vi "Firmware.vi"() -> ()   [LabVIEW 2017]
uses:
  <vilib>/Platform/TimedLoop/XDataNode/timing_clust.ctl
  <vilib>/Platform/TimedLoop/XDataNode/nitl_modes.ctl
  <vilib>/Platform/TimedLoop/XDataNode/wakeup.ctl
  <instrlib>/_niInstr/Instruction Framework/v1/FPGA/Helper Classes/Single Address Space Collection/Single Address Space Collection.lvclass
  C:/Program Files (x86)/National Instruments/LabVIEW 2017/instr.lib/_niInstr/Instruction Framework/v1/FPGA/Interfaces/Address Space Collection/Address Space Collection.lvclass
  <instrlib>/_niInstr/FIFO Register Bus/v1/FPGA/niInstr FIFO Register Bus v1 FPGA.lvclass
  C:/Program Files (x86)/National Instruments/LabVIEW 2017/instr.lib/_niInstr/Instruction Framework/v1/FPGA/Interfaces/Instruction Producer/Instruction Producer.lvclass
  <vilib>/rvi/Emulation/niFpgaGetClockAttributes.vi
  <vilib>/rvi/Emulation/niFpgaSctlEmulationGetInTimedLoop.vi
  <vilib>/rvi/Emulation/niFpgaEmulationReportErrorSimple.vi
  <vilib>/rvi/Emulation/niFpgaProcessEmulError.vi
  <vilib>/rvi/Emulation/niFpgaCriticalErrorInLSC.vi
  <vilib>/rvi/eio/common/nirviEmuTemplateMethod_errors.vi
  <vilib>/eio/EIONode/EIONode.xnode
  <vilib>/Platform/TimedLoop/XDataNode/XDataNode.xnode
  <instrlib>/_niInstr/Instruction Framework/v1/FPGA/Top Level Bus/Register Configuration/Register Configuration.lvclass
  <vilib>/Platform/TimedLoop/XDataNode/XDNodeRunTimeDep.lvlib
  <vilib>/NI/PowerElectronicsControl/ScaleAndLimit/Core/ScaleAndLimit.lvlib
  <vilib>/NI/PowerElectronicsControl/ScaleAndLimit/Core/AddressSpace.lvclass
  <vilib>/NI/PowerElectronicsControl/WaveformAcq/FPGA/WaveformAddressSpace.lvclass
panel:
  out "FaultBuffer":u64 format="%.0x"
  out "LimitsFlag":bool
  out "Sourcing_P1_DI":u16
  out "Sourcing_P0_DI":u16
  out "Sinking_DO":u32 format="%.0x"
  out "Scanned_AI":sgl[](array[numeric])
  out "AO":i16[](array[numeric])
  out "RelayControl_DO":u8 format="%.0x"
  out "LVTTL_DIO":u32 format="%.0x"
  out "HalfBridge":u16 format="%.0x"
  out "TriggerTimestamp":i32
  out "relativeTimestamp":i32
  in  "ManualTrigger":bool
  in  "fifo reg bus ctrl 0":u32
  out "fifo reg bus status 0":u32
  out "fifo reg bus data 0":u64
  out "SimultaneousAILoopRate":u32
  out "Simultaneous_AI":sgl[](array[numeric])
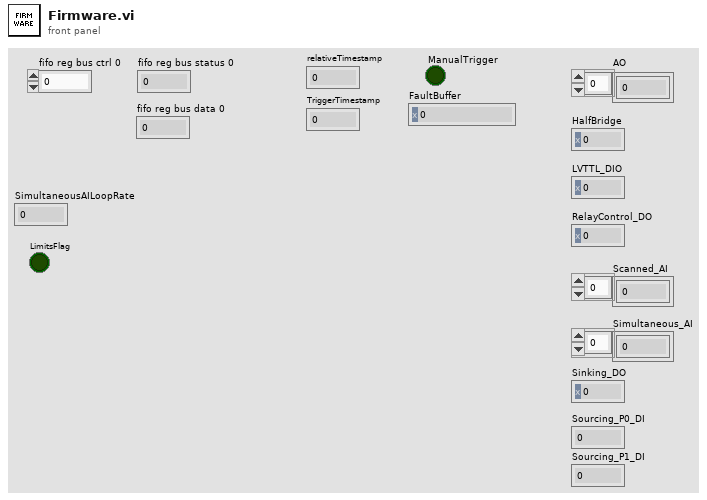
[diagram p1: front panel]
types:
  T1 = typedef "XDNodeRunTimeDep.lvlib/timing_clust.ctl" = cluster{"Expected End [f-1]":u64, "Actual End [f-1]":u64, "Finished Late? [f-1]":bool, "Expected End [i-1]":u64, "Actual End [i-1]":u64, "Finished Late? [i-1]":bool, "Expected Start [i]":u64, "Actual Start [i]":u64, "Expected Start [f]":u64, "Actual Start [f]":u64, "Source Name":string, "Structure Name":string, "Period":i64, "Deadline":i64, "Offset":i64, "Start":i64, "Priority":i32, "Timeout":i32, "Mode":T2, "Wakeup Reason":T3, "Error":errorcluster, "Source Type":string, "Secondary Source Type":string, "Global End Time":u64, "Global Start Time":u64, "Frame Duration":u64, "Iteration Duration":u64, "Assigned CPU":i32, "I/O Scan Engine Mode":u32}
  T2 = typedef "XDNodeRunTimeDep.lvlib/nitl_modes.ctl" = enum32{"No Change", "Process missed periods, maintain original phase", "Discard missed periods, maintain original phase", "Process missed periods, ignore original phase", "Discard missed periods, ignore original phase"}
  T3 = typedef "XDNodeRunTimeDep.lvlib/wakeup.ctl" = enum32{"Normal", "Aborted", "Asynchronous wakeup", "Timing source error", "Timed loop error", "Timeout"}
  T4 = typedef "ScaleAndLimit.lvlib/LimitsRegisters.ctl" = cluster{"HighLimits":refnum<k21>, "LowLimits":refnum<k21>, "ClearLimits":refnum<k21>, "LimitsFlag":refnum<k21>}
  T5 = typedef "ScaleAndLimit.lvlib/ConfigRegisters.ctl" = cluster{"LimitsEnabled":refnum<k21>, "UnscaledHighLimit":refnum<k21>, "UnscaledLowLimit":refnum<k21>, "B":refnum<k21>, "M":refnum<k21>}
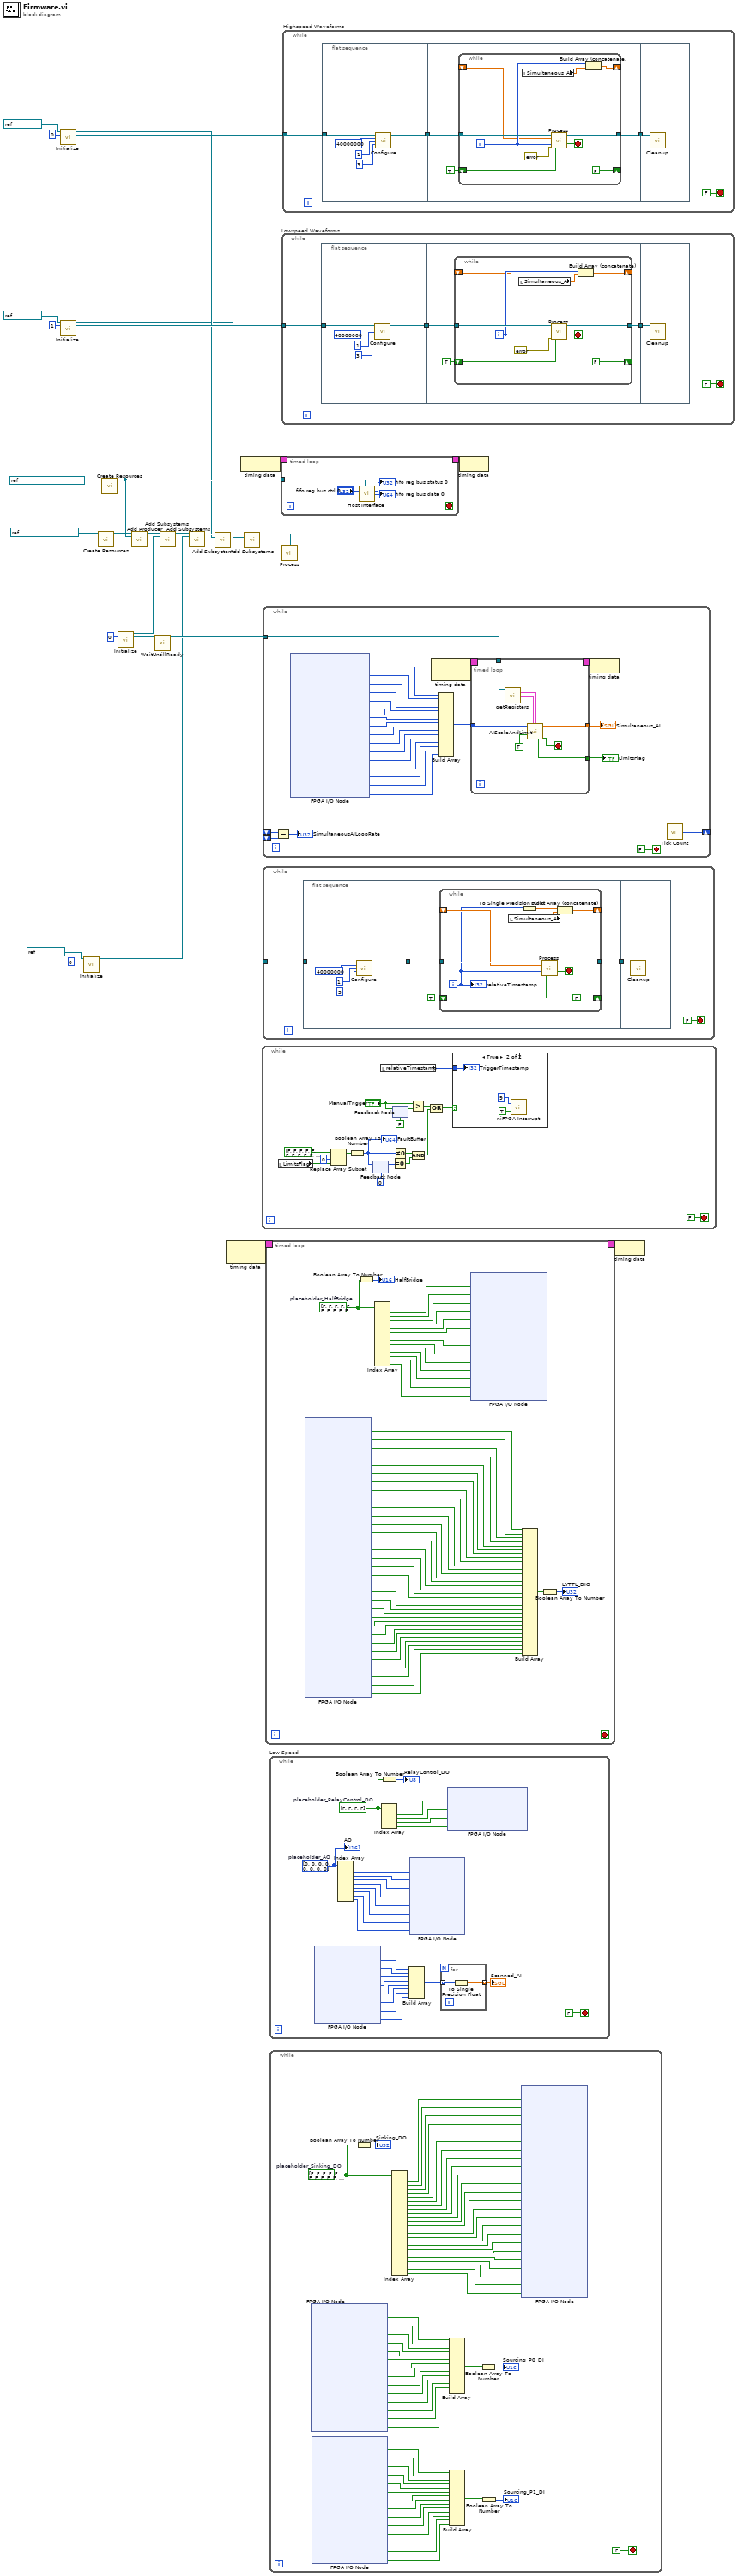
[diagram p0: block diagram]
diagram:
  n1 = call <vilib>:"Initialize.vi"("DMA FIFO"=refnum<k21> "DataSGL0" ("FIFO Out"), "instance"=u8 0) -> ("subsystem"=w3:refnum<class "Single Address Space Collection.lvclass">, "AddressSpace"=w9:refnum<class "WaveformAddressSpace.lvclass">)  [unwired: 12 in]
  n2 = call <vilib>:"Initialize.vi"("DMA FIFO"=refnum<k21> "DataSGL1" ("FIFO Out"), "instance"=u8 1) -> ("subsystem"=w2:refnum<class "Single Address Space Collection.lvclass">, "AddressSpace"=w8:refnum<class "WaveformAddressSpace.lvclass">)  [unwired: 12 in]
  n3 = call <vilib>:"Initialize.vi"("DMA FIFO"=refnum<k21> "DataSGL0" ("FIFO Out"), "instance"=u8 0) -> ("subsystem"=w14:refnum<class "Single Address Space Collection.lvclass">, "AddressSpace"=w16:refnum<class "WaveformAddressSpace.lvclass">)  [unwired: 12 in]
  n4 = call <instrlib>:"Create Resources.vi"("register clock"=refnum<k21> "40 MHz Onboard Clock") -> ("register configuration"=w27:refnum<class "Register Configuration.lvclass">)  [unwired: 14 in]
  n5 = call <instrlib>:"Create Resources.vi"("instruction fifo"=refnum<k21> "reg.host instruction fifo 0") -> ("fifo register bus"=w19:refnum<class "niInstr FIFO Register Bus v1 FPGA.lvclass">)  [unwired: 14 in]
  n6 = call <vilib>:"Initialize.vi"("instance"=u8 0) -> ("subsystem"=w24:refnum<class "Single Address Space Collection.lvclass">, "AddressSpace"=w22:refnum<class "AddressSpace.lvclass">)  [unwired: 13 in]
  n7 = call <instrlib>:"Add Producer.vi"("register configuration in"=w27, "instruction producer"=w19) -> ("register configuration out"=w25:refnum<class "Register Configuration.lvclass">)  [unwired: 13 in]
  n8 = call <vilib>:"WaitUntillReady.vi"("AddressSpace in"=w22) -> ("AddressSpace out"=w21:refnum<class "AddressSpace.lvclass">)  [unwired: 14 in]
  n9 = call <instrlib>:"Add Subsystems.vi"("register configuration in"=w25, "subsystems"=w24) -> ("register configuration out"=w15:refnum<class "Register Configuration.lvclass">)  [unwired: 13 in]
  n10 = call <instrlib>:"Add Subsystems.vi"("register configuration in"=w15, "subsystems"=w14) -> ("register configuration out"=w4:refnum<class "Register Configuration.lvclass">)  [unwired: 13 in]
  n11 = call <instrlib>:"Add Subsystems.vi"("register configuration in"=w4, "subsystems"=w3) -> ("register configuration out"=w5:refnum<class "Register Configuration.lvclass">)  [unwired: 13 in]
  n12 = node-c288() -> (w13:T1)  [unwired: 1 in]
  n13 = node-c288() -> (w29:T1)
  n14 = call <instrlib>:"Add Subsystems.vi"("register configuration in"=w5, "subsystems"=w2) -> ("register configuration out"=w1:refnum<class "Register Configuration.lvclass">)  [unwired: 13 in]
  n15 = while {
    stop <- FALSE stop-if-true
    n16 = local read "LimitsFlag"() -> (w38:bool)
    n17 = Replace Array Subset(array=bool[] [FALSE, FALSE, FALSE, FALSE, FALSE, FALSE, FALSE, FALSE, FALSE, FALSE, FALSE, FALSE, FALSE, FALSE, FALSE, FALSE, FALSE, FALSE, FALSE, FALSE, FALSE, FALSE, FALSE, FALSE, FALSE, FALSE, FALSE, FALSE, FALSE, FALSE, FALSE, FALSE, FALSE, FALSE, FALSE, FALSE, FALSE, FALSE, FALSE, FALSE, FALSE, FALSE, FALSE, FALSE, FALSE, FALSE, FALSE, FALSE, FALSE, FALSE, FALSE, FALSE, FALSE, FALSE, FALSE, FALSE, FALSE, FALSE, FALSE, FALSE, FALSE, FALSE, FALSE, FALSE], new element=w38, index=0) -> (w36:bool[])
    n18 = Boolean Array To Number(Boolean array=w36) -> (number=w34:u64)
    "FaultBuffer" <- w34
    n19 = feedback-in #1(w34) -> ()
    n20 = feedback #1(u64 0) -> (w33:u64)
    n21 = local read "relativeTimestamp"() -> (w40:i32)
    n22 = feedback-in #2("ManualTrigger") -> ()
    n23 = feedback #2(FALSE ("ManualTrigger")) -> (w44:bool)
    n24 = Equal To 0?(x=w33) -> (x = 0?=w31:bool)
    n25 = Not Equal To 0?(x=w34) -> (x != 0?=w32:bool)
    n26 = Greater?(x="ManualTrigger", y=w44) -> (0:w45:bool)
    n27 = Compound Arithmetic op=AND(w32, w31) -> (w30:bool)
    n28 = Compound Arithmetic op=OR(w45, w30) -> (w42:bool)
    n29 = case shown="True" w42 {
      tunnel: w40 -> [_ w47]
      frame False {
      }
      frame True {
        n30 = call <vilib>:"niFPGA Interrupt.vi"("Wait Until Cleared (F)"=TRUE, "IRQ Number (0)"=u8 9) -> ()  [unwired: 1 in]
        "TriggerTimestamp" <- w47
      }
    }
  }
  n31 = while {
    shift-right: [w75] -> _
    shift-left: _ -> [w74]
    shift-left: _ -> [w73]
    tunnel: w21 -> [w53]
    stop <- FALSE stop-if-true
    n32 = Subtract(x=w74, y=w73) -> (x-y=→"SimultaneousAILoopRate":u32)
    n33 = xnode "FPGA I/O Node"() -> ("RMC/Simultaneous/AI0"=w71:i16, "RMC/Simultaneous/AI1"=w70:i16, "RMC/Simultaneous/AI2"=w69:i16, "RMC/Simultaneous/AI3"=w68:i16, "RMC/Simultaneous/AI4"=w67:i16, "RMC/Simultaneous/AI5"=w66:i16, "RMC/Simultaneous/AI6"=w65:i16, "RMC/Simultaneous/AI7"=w64:i16, "RMC/Simultaneous/AI8"=w63:i16, "RMC/Simultaneous/AI9"=w62:i16, "RMC/Simultaneous/AI10"=w61:i16, "RMC/Simultaneous/AI11"=w60:i16, "RMC/Simultaneous/AI12"=w59:i16, "RMC/Simultaneous/AI13"=w58:i16, "RMC/Simultaneous/AI14"=w57:i16, "RMC/Simultaneous/AI15"=w51:i16)  [unwired: 16 in, 16 out]
    n34 = node-c288() -> (w56:T1)  [unwired: 1 in]
    n35 = Build Array(w71, w70, w69, w68, w67, w66, w65, w64, w63, w62, w61, w60, w59, w58, w57, w51) -> (w52:i16[])
    n36 = timed-loop {
      timing: w56 -> [_]
      timing-out: [_] -> w55
      tunnel: w52 -> [w84]
      tunnel: [w82] -> w54
      tunnel: w53 -> [w80]
      tunnel: [w77] -> w50
      stop <- w81 stop-if-true
      n37 = call <vilib>:"getRegisters.vi"("AddressSpace in"=w80) -> ("LimitsRegisters"=w78:T4, "ConfigRegisters"=w79:T5)  [unwired: 12 in, 1 out]
      n38 = call <vilib>:"AIScaleAndLimit.vi"("UnscaledAI"=w84, "ConfigRegisters"=w79, "LimitsRegisters"=w78, "input valid"=TRUE) -> ("ScaledAI"=w82:sgl[], "LimitsFlag"=w77:bool, "output valid"=w81:bool)  [unwired: 6 in, 3 out]
    }
    "Simultaneous_AI" <- w54
    "LimitsFlag" <- w50
    n39 = node-c288(w55) -> ()
    n40 = call "Tick Count"() -> ("Tick Count(Ticks)"=w75:u32)
  }
  n41 = while {
    tunnel: w16 -> [w89]
    stop <- FALSE stop-if-true
    n42 = flat-sequence {
      tunnel: [w93] -> w91
      tunnel: w89 -> [w94]
      tunnel: w91 -> [w100]
      tunnel: [w99] -> w90
      tunnel: w90 -> [w111]
      frame #0 {
        n43 = call <vilib>:"Configure.vi"("WaveformAddressSpace in"=w94, "oclk_freq"=u32 40000000, "oclk_mult"=u32 1, "UnderflowMargin"=u32 3 ("y")) -> ("WaveformAddressSpace out"=w93:refnum<class "WaveformAddressSpace.lvclass">)  [unwired: 11 in]
      }
      frame #1 {
        n44 = while {
          shift-right: [w109] -> _
          shift-left: _ -> [w103]
          shift-right: [FALSE] -> _
          shift-left: TRUE -> [w105]
          tunnel: w100 -> [w107]
          tunnel: [w106] -> w99
          i -> [w102]
          stop <- w108 stop-if-true
          n45 = local read "Simultaneous_AI"() -> (w104:sgl[])
          n46 = To Single Precision Float(number=w102) -> (single precision float=w101:sgl)
          n47 = call <instrlib>:"Process.vi"("WaveformAddressSpace in"=w107, "Data"=w103, "Iteration"=w102, "FirstIteration"=w105) -> ("WaveformAddressSpace out"=w106:refnum<class "WaveformAddressSpace.lvclass">, "stop"=w108:bool)  [unwired: 8 in, 2 out]
          n48 = Build Array (concatenate)(w101, w104) -> (w109:sgl[])
          "relativeTimestamp" <- w102
        }
      }
      frame #2 {
        n49 = call <vilib>:"Cleanup.vi"("WaveformAddressSpace in"=w111) -> ()  [unwired: 14 in, 1 out]
      }
    }
  }
  n50 = timed-loop {
    timing: w13 -> [_]
    timing-out: [_] -> w12
    stop <- _ stop-if-true
    w147 = bool[] [FALSE, FALSE, FALSE, FALSE, FALSE, FALSE, FALSE, FALSE, FALSE, FALSE, FALSE, FALSE, FALSE, FALSE]  # placeholder_HalfBridge
    n51 = xnode "FPGA I/O Node"() -> ("RMC/LVTTL/DIO0"=w145:bool, "RMC/LVTTL/DIO1"=w144:bool, "RMC/LVTTL/DIO2"=w143:bool, "RMC/LVTTL/DIO3"=w142:bool, "RMC/LVTTL/DIO4"=w141:bool, "RMC/LVTTL/DIO5"=w140:bool, "RMC/LVTTL/DIO6"=w139:bool, "RMC/LVTTL/DIO7"=w138:bool, "RMC/LVTTL/DIO8"=w137:bool, "RMC/LVTTL/DIO9"=w136:bool, "RMC/LVTTL/DIO10"=w135:bool, "RMC/LVTTL/DIO11"=w134:bool, "RMC/LVTTL/DIO12"=w133:bool, "RMC/LVTTL/DIO13"=w132:bool, "RMC/LVTTL/DIO14"=w131:bool, "RMC/LVTTL/DIO15"=w130:bool, "RMC/LVTTL/DIO16"=w129:bool, "RMC/LVTTL/DIO17"=w128:bool, "RMC/LVTTL/DIO18"=w127:bool, "RMC/LVTTL/DIO19"=w126:bool, "RMC/LVTTL/DIO20"=w125:bool, "RMC/LVTTL/DIO21"=w124:bool, "RMC/LVTTL/DIO22"=w123:bool, "RMC/LVTTL/DIO23"=w122:bool, "RMC/LVTTL/DIO24"=w121:bool, "RMC/LVTTL/DIO25"=w120:bool, "RMC/LVTTL/DIO26"=w119:bool, "RMC/LVTTL/DIO27"=w118:bool, "RMC/LVTTL/DIO28"=w117:bool, "RMC/LVTTL/DIO29"=w116:bool, "RMC/LVTTL/DIO30"=w115:bool, "RMC/LVTTL/DIO31"=w114:bool)  [unwired: 32 in, 32 out]
    n52 = Boolean Array To Number(Boolean array=w147) -> (number=→"HalfBridge":u16)
    n53 = Index Array(array=w147) -> (element #1=w161:bool, element #2=w160:bool, element #3=w159:bool, element #4=w158:bool, element #5=w157:bool, element #6=w156:bool, element #7=w155:bool, element #8=w154:bool, element #9=w153:bool, element #10=w152:bool, element #11=w151:bool, element #12=w150:bool, element #13=w149:bool, element #14=w148:bool)  [unwired: 14 in]
    n54 = xnode "FPGA I/O Node"("RMC/Half-Bridge/DO0"=w161, "RMC/Half-Bridge/DO1"=w160, "RMC/Half-Bridge/DO2"=w159, "RMC/Half-Bridge/DO3"=w158, "RMC/Half-Bridge/DO4"=w157, "RMC/Half-Bridge/DO5"=w156, "RMC/Half-Bridge/DO6"=w155, "RMC/Half-Bridge/DO7"=w154, "RMC/Half-Bridge/DO8"=w153, "RMC/Half-Bridge/DO9"=w152, "RMC/Half-Bridge/DO10"=w151, "RMC/Half-Bridge/DO11"=w150, "RMC/Half-Bridge/DO12"=w149, "RMC/Half-Bridge/DO13"=w148) -> ()  [unwired: 14 in, 14 out]
    n55 = Build Array(w145, w144, w143, w142, w141, w140, w139, w138, w137, w136, w135, w134, w133, w132, w131, w130, w129, w128, w127, w126, w125, w124, w123, w122, w121, w120, w119, w118, w117, w116, w115, w114) -> (w113:bool[])
    n56 = Boolean Array To Number(Boolean array=w113) -> (number=→"LVTTL_DIO":u32)
  }
  n57 = while "Low Speed" {
    stop <- FALSE stop-if-true
    w175 = bool[] [FALSE, FALSE, FALSE, FALSE]  # placeholder_RelayControl_DO
    w188 = i16[] [0, 0, 0, 0, 0, 0, 0, 0]  # placeholder_AO
    n58 = xnode "FPGA I/O Node"() -> ("RMC/Scanned/AI0"=w173:i16, "RMC/Scanned/AI1"=w172:i16, "RMC/Scanned/AI2"=w171:i16, "RMC/Scanned/AI3"=w170:i16, "RMC/Scanned/AI4"=w169:i16, "RMC/Scanned/AI5"=w168:i16, "RMC/Scanned/AI6"=w167:i16, "RMC/Scanned/AI7"=w166:i16)  [unwired: 8 in, 8 out]
    n59 = Index Array(array=w188) -> (element #1=w187:i16, element #2=w186:i16, element #3=w185:i16, element #4=w184:i16, element #5=w183:i16, element #6=w182:i16, element #7=w181:i16, element #8=w180:i16)  [unwired: 8 in]
    n60 = Boolean Array To Number(Boolean array=w175) -> (number=→"RelayControl_DO":u8)
    n61 = Index Array(array=w175) -> (element #1=w179:bool, element #2=w178:bool, element #3=w177:bool, element #4=w176:bool)  [unwired: 4 in]
    n62 = Build Array(w173, w172, w171, w170, w169, w168, w167, w166) -> (w165:i16[])
    n63 = xnode "FPGA I/O Node"("RMC/AO/AO0"=w187, "RMC/AO/AO1"=w186, "RMC/AO/AO2"=w185, "RMC/AO/AO3"=w184, "RMC/AO/AO4"=w183, "RMC/AO/AO5"=w182, "RMC/AO/AO6"=w181, "RMC/AO/AO7"=w180) -> ()  [unwired: 8 in, 8 out]
    n64 = for {
      tunnel: w165 -> [w191] mode=indexing
      tunnel: [w190] -> w164 mode=indexing
      n65 = To Single Precision Float(number=w191) -> (single precision float=w190:sgl)
    }
    "Scanned_AI" <- w164
    n66 = xnode "FPGA I/O Node"("RMC/Relay Control/DO0"=w179, "RMC/Relay Control/DO1"=w178, "RMC/Relay Control/DO2"=w177, "RMC/Relay Control/DO3"=w176) -> ()  [unwired: 4 in, 4 out]
    "AO" <- w188
  }
  n67 = while {
    stop <- FALSE stop-if-true
    w249 = bool[] [FALSE, FALSE, FALSE, FALSE, FALSE, FALSE, FALSE, FALSE, FALSE, FALSE, FALSE, FALSE, FALSE, FALSE, FALSE, FALSE, FALSE, FALSE, FALSE, FALSE, FALSE, FALSE, FALSE, FALSE]  # placeholder_Sinking_DO
    n68 = xnode "FPGA I/O Node"() -> ("RMC/Sourcing P0/DI0"=w223:bool, "RMC/Sourcing P0/DI1"=w222:bool, "RMC/Sourcing P0/DI2"=w221:bool, "RMC/Sourcing P0/DI3"=w220:bool, "RMC/Sourcing P0/DI4"=w219:bool, "RMC/Sourcing P0/DI5"=w218:bool, "RMC/Sourcing P0/DI6"=w217:bool, "RMC/Sourcing P0/DI7"=w216:bool, "RMC/Sourcing P0/DI8"=w215:bool, "RMC/Sourcing P0/DI9"=w214:bool, "RMC/Sourcing P0/DI10"=w213:bool, "RMC/Sourcing P0/DI11"=w212:bool, "RMC/Sourcing P0/DI12"=w211:bool, "RMC/Sourcing P0/DI13"=w210:bool)  [unwired: 14 in, 14 out]
    n69 = xnode "FPGA I/O Node"() -> ("RMC/Sourcing P1/DI0"=w192:bool, "RMC/Sourcing P1/DI1"=w193:bool, "RMC/Sourcing P1/DI2"=w194:bool, "RMC/Sourcing P1/DI3"=w195:bool, "RMC/Sourcing P1/DI4"=w196:bool, "RMC/Sourcing P1/DI5"=w197:bool, "RMC/Sourcing P1/DI6"=w198:bool, "RMC/Sourcing P1/DI7"=w199:bool, "RMC/Sourcing P1/DI8"=w200:bool, "RMC/Sourcing P1/DI9"=w201:bool, "RMC/Sourcing P1/DI10"=w202:bool, "RMC/Sourcing P1/DI11"=w203:bool, "RMC/Sourcing P1/DI12"=w204:bool, "RMC/Sourcing P1/DI13"=w205:bool)  [unwired: 14 in, 14 out]
    n70 = Boolean Array To Number(Boolean array=w249) -> (number=→"Sinking_DO":u32)
    n71 = Index Array(array=w249) -> (element #1=w248:bool, element #2=w247:bool, element #3=w246:bool, element #4=w245:bool, element #5=w244:bool, element #6=w243:bool, element #7=w242:bool, element #8=w241:bool, element #9=w240:bool, element #10=w239:bool, element #11=w238:bool, element #12=w237:bool, element #13=w236:bool, element #14=w235:bool, element #15=w234:bool, element #16=w233:bool, element #17=w232:bool, element #18=w231:bool, element #19=w230:bool, element #20=w229:bool, element #21=w228:bool, element #22=w227:bool, element #23=w226:bool, element #24=w225:bool)  [unwired: 24 in]
    n72 = Build Array(w223, w222, w221, w220, w219, w218, w217, w216, w215, w214, w213, w212, w211, w210) -> (w209:bool[])
    n73 = Build Array(w192, w193, w194, w195, w196, w197, w198, w199, w200, w201, w202, w203, w204, w205) -> (w206:bool[])
    n74 = Boolean Array To Number(Boolean array=w209) -> (number=→"Sourcing_P0_DI":u16)
    n75 = Boolean Array To Number(Boolean array=w206) -> (number=→"Sourcing_P1_DI":u16)
    n76 = xnode "FPGA I/O Node"("RMC/Sinking/DO0"=w248, "RMC/Sinking/DO1"=w247, "RMC/Sinking/DO2"=w246, "RMC/Sinking/DO3"=w245, "RMC/Sinking/DO4"=w244, "RMC/Sinking/DO5"=w243, "RMC/Sinking/DO6"=w242, "RMC/Sinking/DO7"=w241, "RMC/Sinking/DO8"=w240, "RMC/Sinking/DO9"=w239, "RMC/Sinking/DO10"=w238, "RMC/Sinking/DO11"=w237, "RMC/Sinking/DO12"=w236, "RMC/Sinking/DO13"=w235, "RMC/Sinking/DO14"=w234, "RMC/Sinking/DO15"=w233, "RMC/Sinking/DO16"=w232, "RMC/Sinking/DO17"=w231, "RMC/Sinking/DO18"=w230, "RMC/Sinking/DO19"=w229, "RMC/Sinking/DO20"=w228, "RMC/Sinking/DO21"=w227, "RMC/Sinking/DO22"=w226, "RMC/Sinking/DO23"=w225) -> ()  [unwired: 24 in, 24 out]
  }
  n77 = timed-loop {
    timing: w29 -> [_]
    timing-out: [_] -> w28
    tunnel: w19 -> [w254]
    stop <- _ stop-if-true
    n78 = call <instrlib>:"Host Interface.vi"("fifo register bus"=w254, "fifo reg bus ctrl 0"="fifo reg bus ctrl 0") -> ("fifo reg bus status 0"=→"fifo reg bus status 0":u32, "fifo reg bus data 0"=→"fifo reg bus data 0":u64)  [unwired: 12 in]
  }
  n79 = while "Lowspeed Waveforms" {
    tunnel: w8 -> [w257]
    stop <- FALSE stop-if-true
    n80 = flat-sequence {
      tunnel: [w261] -> w259
      tunnel: w257 -> [w262]
      tunnel: w259 -> [w268]
      tunnel: [w267] -> w258
      tunnel: w258 -> [w279]
      frame #0 {
        n81 = call <vilib>:"Configure.vi"("WaveformAddressSpace in"=w262, "oclk_freq"=u32 40000000, "oclk_mult"=u32 1, "UnderflowMargin"=u32 3 ("y")) -> ("WaveformAddressSpace out"=w261:refnum<class "WaveformAddressSpace.lvclass">)  [unwired: 11 in]
      }
      frame #1 {
        n82 = while {
          shift-right: [w277] -> _
          shift-left: _ -> [w269]
          shift-right: [FALSE] -> _
          shift-left: TRUE -> [w272]
          tunnel: w268 -> [w274]
          tunnel: [w273] -> w267
          i -> [w271]
          stop <- w275 stop-if-true
          n83 = local read "Simultaneous_AI"() -> (w270:sgl[])
          n84 = call <instrlib>:"Process.vi"("WaveformAddressSpace in"=w274, "Data"=w269, "Iteration"=w271, "error in (no error)"=errorcluster {"status"=FALSE, "code"=0, "source"=""} ("injectError1"), "FirstIteration"=w272) -> ("WaveformAddressSpace out"=w273:refnum<class "WaveformAddressSpace.lvclass">, "stop"=w275:bool)  [unwired: 7 in, 2 out]
          n85 = Build Array (concatenate)(w271, w270) -> (w277:sgl[])
        }
      }
      frame #2 {
        n86 = call <vilib>:"Cleanup.vi"("WaveformAddressSpace in"=w279) -> ()  [unwired: 14 in, 1 out]
      }
    }
  }
  n87 = call <instrlib>:"Process.vi"("register configuration"=w1) -> ()  [unwired: 15 in]
  n88 = while "Highspeed Waveforms" {
    tunnel: w9 -> [w280]
    stop <- FALSE stop-if-true
    n89 = flat-sequence {
      tunnel: [w284] -> w282
      tunnel: w280 -> [w285]
      tunnel: w282 -> [w291]
      tunnel: [w290] -> w281
      tunnel: w281 -> [w302]
      frame #0 {
        n90 = call <vilib>:"Configure.vi"("WaveformAddressSpace in"=w285, "oclk_freq"=u32 40000000, "oclk_mult"=u32 1, "UnderflowMargin"=u32 3 ("y")) -> ("WaveformAddressSpace out"=w284:refnum<class "WaveformAddressSpace.lvclass">)  [unwired: 11 in]
      }
      frame #1 {
        n91 = while {
          shift-right: [w300] -> _
          shift-left: _ -> [w293]
          shift-right: [FALSE] -> _
          shift-left: TRUE -> [w296]
          tunnel: w291 -> [w298]
          tunnel: [w297] -> w290
          i -> [w295]
          stop <- w299 stop-if-true
          n92 = local read "Simultaneous_AI"() -> (w294:sgl[])
          n93 = call <instrlib>:"Process.vi"("WaveformAddressSpace in"=w298, "Data"=w293, "Iteration"=w295, "error in (no error)"=errorcluster {"status"=FALSE, "code"=0, "source"=""}, "FirstIteration"=w296) -> ("WaveformAddressSpace out"=w297:refnum<class "WaveformAddressSpace.lvclass">, "stop"=w299:bool)  [unwired: 7 in, 2 out]
          n94 = Build Array (concatenate)(w295, w294) -> (w300:sgl[])
        }
      }
      frame #2 {
        n95 = call <vilib>:"Cleanup.vi"("WaveformAddressSpace in"=w302) -> ()  [unwired: 14 in, 1 out]
      }
    }
  }
  n96 = node-c288(w28) -> ()
  n97 = node-c288(w12) -> ()
